vi "Handle Errors.vi"(8 "error in":errorcluster, 11 "nCRD in":refnum<class "gCRD.lvclass">) -> (0 "error out":errorcluster, 2 "errors":errorcluster[](array[cluster]), 3 "nCRD out":refnum<class "gCRD.lvclass">)   [LabVIEW 2017, in "gCRDS.lvlib" / "gCRD.lvclass"]
uses:
  gCRD.lvclass
  <vilib>/MSR Consulting, LLC/General Reuse/CRDS/Main/CRDS.lvclass
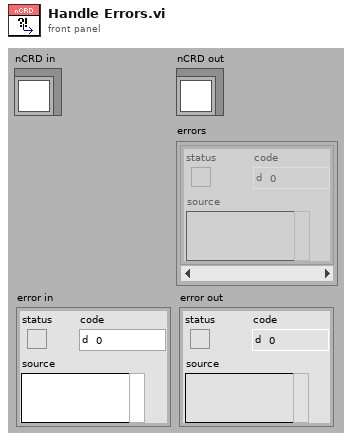
[diagram p1: front panel]
types:
  T1 = typedef "FPGA Ref.ctl" = refnum<k20>
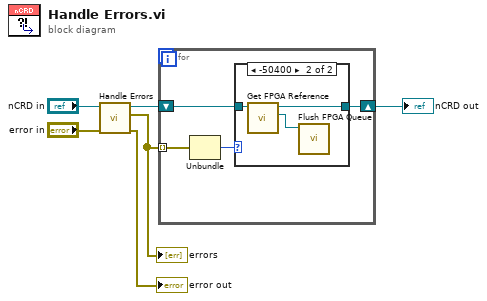
[diagram p0: block diagram]
diagram:
  n1 = call-parent "Handle Errors.vi"("error in"="error in", "Instrument in"="nCRD in") -> ("error out"=→"error out":errorcluster, "errors"=w3:errorcluster[], "Instrument out"=w2:refnum<class "gCRD.lvclass">)  [unwired: 7 in]
  "errors" <- w3
  n2 = for {
    tunnel: w3 -> [w10] mode=indexing
    shift-right: [w8] -> w1
    shift-left: w2 -> [w9]
    n3 = Unbundle(w10) -> ("code"=w7:i32)  [unwired: 2 out]
    n4 = case shown="-50400" w7 {
      tunnel: w9 -> [w11 w14]
      tunnel: [w11 w13] -> w8
      frame 0, Default {
      }
      frame -50400 {
        n5 = call "Get FPGA Reference.vi"("nCRD in"=w14) -> ("FPGA Ref"=w12:T1, "nCRD out"=w13:refnum<class "gCRD.lvclass">)  [unwired: 8 in, 1 out]
        n6 = call "Flush FPGA Queue.vi"("Refnum in"=w12) -> ()  [unwired: 10 in, 1 out]
      }
    }
  }
  "nCRD out" <- w1
